vi "Read Data.vi"   [LabVIEW 2013, in "Keithley 27XX.lvlib"]
doc: "This VI performs various types of reads to acquire measurement data."
uses:
  <instrlib>/Keithley 27XX/Keithley 27XX.lvlib
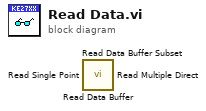
[diagram p0: block diagram]
diagram:
  n1 = call <instrlib>:"Read Data Buffer.vi"() -> ()  [unwired: 10 in, 6 out]
  n2 = call <instrlib>:"Read Data Buffer Subset.vi"() -> ()  [unwired: 10 in, 6 out]
  n3 = call <instrlib>:"Read Single Point.vi"() -> ()  [unwired: 13 in, 3 out]
  n4 = call <instrlib>:"Read Multiple Direct.vi"() -> ()  [unwired: 10 in, 6 out]
